vi "Model 3566-Set Online.vi"(8 "error in":errorcluster, 10 "Online?":bool, 11 "Model 3566 Setting In":T1) -> (0 "error out":errorcluster, 2 "Respond":string, 3 "Model 3566 Setting Out":T1)   [LabVIEW 2018]
uses:
  Data Def/Model 3566-Setting.ctl
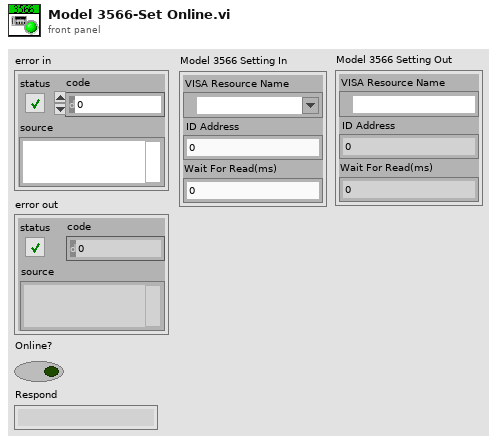
[diagram p1: front panel]
types:
  T1 = typedef "Model 3566-Setting.ctl" = cluster{"VISA Resource Name":refnum<visa-resource-name>, "ID Address":u8, "Wait For Read(ms)":u32}
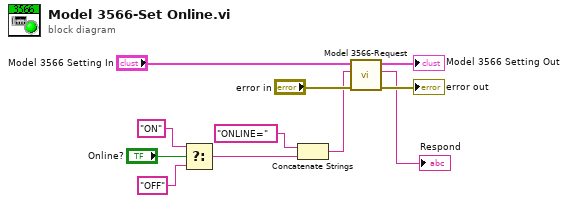
[diagram p0: block diagram]
diagram:
  n1 = Select(t="ON" ("write buffer"), s="Online?", f="OFF" ("write buffer")) -> (s? t:f=w7:string)
  n2 = Concatenate Strings("ONLINE=" ("write buffer"), w7) -> (w4:string)
  n3 = call "Model 3566-Request.vi"("error in"="error in", "Command"=w4, "Model 3566 Setting In"="Model 3566 Setting In") -> ("error out"=→"error out":errorcluster, "Respond"=→"Respond":string, "Model 3566 Setting Out"=→"Model 3566 Setting Out":T1)  [unwired: 6 in]
